vi "img.BGFF.vi"(6 "DVR":T1, 9 "image in":u16[][](array[numeric])) -> (1 "image out":u16[][](array[numeric]))   [LabVIEW 2020]
uses:
  _controls/data.ref.ctl
  _controls/state.ctl
  _controls/data.vars.ctl
  _controls/data.ctl
  _controls/flip.ctl
  <vilib>/vision/Image Controls.llb/IMAQ Image.ctl
  camera/camera.lvclass
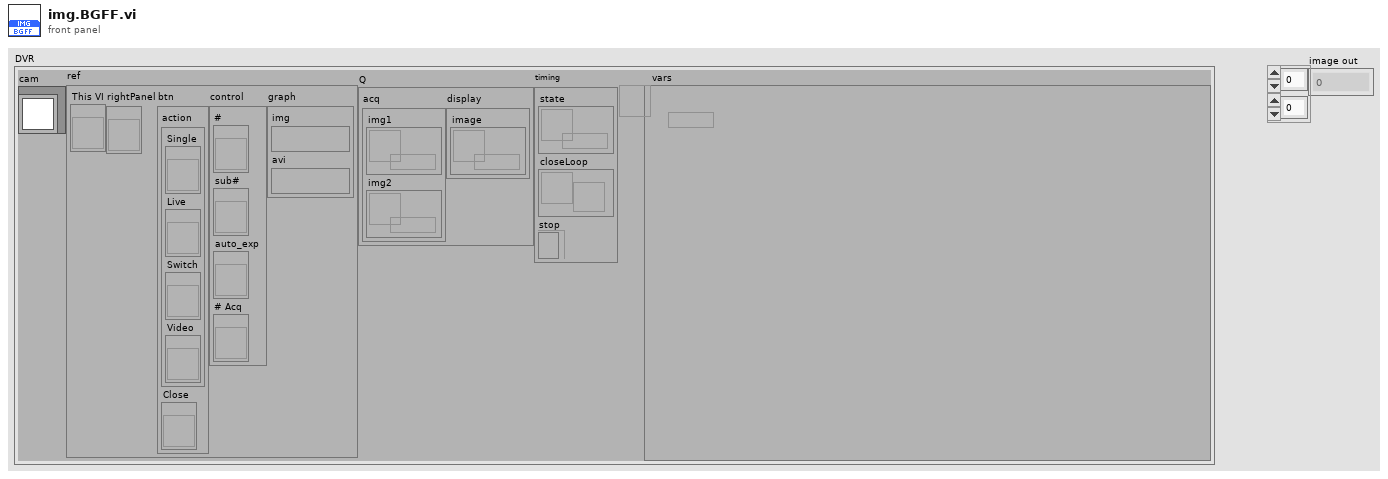
[diagram p1: front panel]
types:
  T1 = typedef "data.ctl" = cluster{"cam":refnum<class "camera.lvclass">, "ref":T2, "Q":cluster{"acq":cluster{"img1":refnum<queue>, "img2":refnum<queue>}, "display":cluster{"image":refnum<queue>}}, "timing":cluster{"state":refnum<queue>, "closeLoop":refnum<notifier>, "stop":refnum<k4>}, "vars":refnum<data-value>}
  T2 = typedef "data.ref.ctl" = cluster{"This VI":refnum<vi>, "rightPanel":refnum<vi>, "btn":cluster{"action":cluster{"Single":refnum<vi>, "Live":refnum<vi>, "Switch":refnum<vi>, "Video":refnum<vi>}, "Close":refnum<vi>}, "control":cluster{"#":refnum<vi>, "sub#":refnum<vi>, "auto_exp":refnum<vi>, "# Acq":refnum<vi>}, "graph":cluster{"img":T3, "avi":T3}}
  T3 = typedef "IMAQ Image.ctl" = refnum<image>
  T4 = typedef "data.vars.ctl" = cluster{"save":cluster{"base_folder":cluster{"Folder":path, "tif":bool, "jpg":bool}, "module":string, "#":u32, "sub#":u8, "save.op":enum16{"Full", "Light"}, "same?":bool, "Shift":enum16{"Single", "Leapfrog"}, "jpg?":bool, "flip":T5}, "acq":cluster{"# Acq":u16, "rotate":bool, "FPS":dbl}, "calib.manual":cluster{"BG":cluster{"Image":u16[][], "enabled?":bool}, "FF":cluster{"Image":u16[][], "enabled?":bool}}}
  T5 = typedef "flip.ctl" = cluster{"x":bool, "y":bool}
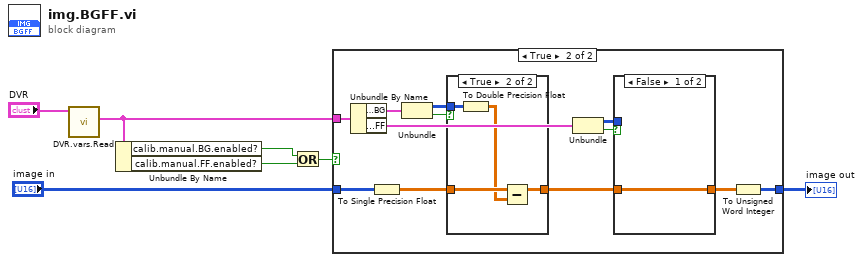
[diagram p0: block diagram]
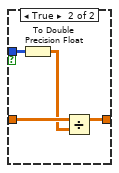
[diagram p3: hidden frame]
diagram:
  n1 = call "DVR.vars.Read.vi"("DVR.state"="DVR") -> ("vars"=w4:T4)  [unwired: 9 in, 1 out]
  n2 = Unbundle By Name(w4) -> ("calib.manual.BG.enabled?"=w3:bool, "calib.manual.FF.enabled?"=w2:bool)
  n3 = Or(x=w3, y=w2) -> (x .or. y?=w1:bool)
  n4 = case shown="True" w1 {
    tunnel: "image in" -> [w8 w20]
    tunnel: w4 -> [_ w18]
    tunnel: [w8 w9] -> w5
    frame False {
    }
    frame True {
      n5 = Unbundle By Name(w18) -> ("calib.manual.BG"=w17:cluster{"Image":u16[][], "enabled?":bool}, "calib.manual.FF"=w14:cluster{"Image":u16[][], "enabled?":bool})
      n6 = To Single Precision Float(number=w20) -> (single precision float=w19:sgl[][])
      n7 = Unbundle(w17) -> ("Image"=w16:u16[][], "enabled?"=w15:bool)
      n8 = case shown="True" w15 {
        tunnel: w19 -> [w26 w30]
        tunnel: [w26 w29] -> w11
        tunnel: w16 -> [_ w28]
        frame False {
        }
        frame True {
          n9 = To Double Precision Float(number=w28) -> (double precision float=w27:dbl[][])
          n10 = Subtract(x=w30, y=w27) -> (x-y=w29:dbl[][])
        }
      }
      n11 = Unbundle(w14) -> ("Image"=w12:u16[][], "enabled?"=w13:bool)
      n12 = case shown="False" w13 {
        tunnel: w11 -> [w21 w25]
        tunnel: [w21 w24] -> w10
        tunnel: w12 -> [_ w23]
        frame False {
        }
        frame True {
          n13 = To Double Precision Float(number=w23) -> (double precision float=w22:dbl[][])
          n14 = Divide(x=w25, y=w22) -> (x/y=w24:dbl[][])
        }
      }
      n15 = To Unsigned Word Integer(number=w10) -> (unsigned 16bit integer=w9:u16[][])
    }
  }
  "image out" <- w5
